vi "Complete PWM V2.vi"() -> ()   [LabVIEW 2023]
uses:
  <vilib>/Utility/error.llb/DialogType.ctl
  <vilib>/DAQmx/write.llb/DAQmx Write (Counter Frequency 1Chan 1Samp).vi
  <vilib>/DAQmx/create/channels.llb/DAQmx Create Channel (CO-Pulse Generation-Frequency).vi
  <vilib>/DAQmx/configure/timing.llb/DAQmx Timing (Implicit).vi
  <vilib>/DAQmx/miscellaneous.llb/DAQmx Fill In Error Info.vi
panel:
  out "OUT Gate":bool
  out "IN Gate":bool
  in  "stop":bool
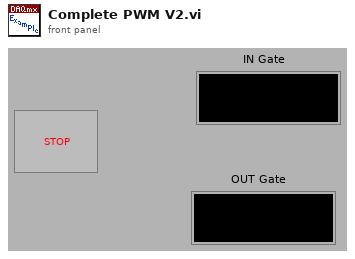
[diagram p1: front panel]
types:
  T1 = typedef "DialogType.ctl" = u16
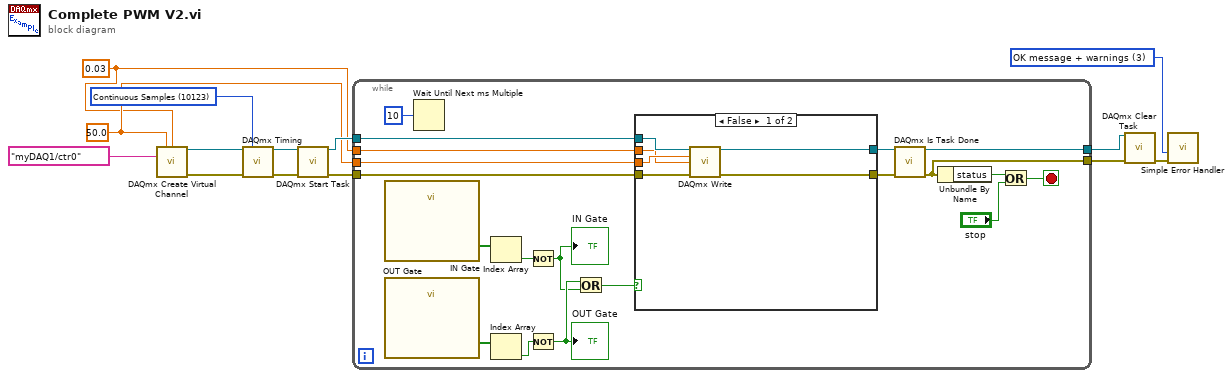
[diagram p0: block diagram]
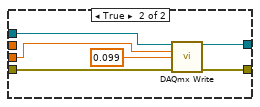
[diagram p2: hidden frame]
diagram:
  w1 = 0.03 ("Duty Cycle")
  w2 = 50.0 ("Frequency")
  w3 = T1 3 items=["no dialog", "OK message", "continue or stop message", "OK message + warnings", "continue/stop + warnings"] ("type of dialog (OK msg:1)")
  w6 = 10123 items=["Finite Samples"=10178, "Continuous Samples"=10123] ("sample mode")
  n1 = call-poly <vilib>:"DAQmx Create Virtual Channel.vi"("frequency"=w2, "duty cycle"=w1, "counter"=tag "myDAQ1/ctr0" ("Counter(s)")) -> ("task out"=w11:refnum<k21>, "error out"=w14:errorcluster)  [unwired: 11 in]
  n2 = call-poly <vilib>:"DAQmx Timing.vi"("task/channels in"=w11, "sample mode"=w6, "error in"=w14) -> ("task out"=w7:refnum<k21>, "error out"=w8:errorcluster)  [unwired: 11 in]
  n3 = call <vilib>:"DAQmx Start Task.vi"("task/channels in"=w7, "error in"=w8) -> ("task out"=w10:refnum<k21>, "error out"=w13:errorcluster)  [unwired: 12 in]
  n4 = while {
    tunnel: w13 -> [w25]
    tunnel: w10 -> [w26]
    tunnel: [w33] -> w9
    tunnel: [w32] -> w4
    tunnel: w2 -> [w24]
    tunnel: w1 -> [w15]
    stop <- w31 stop-if-true
    n5 = call "IN Gate"() -> ("data"=w22:bool[])  [unwired: 17 in, 2 out]
    n6 = call "OUT Gate"() -> ("data"=w20:bool[])  [unwired: 17 in, 2 out]
    n7 = Wait Until Next ms Multiple(millisecond multiple=u32 10) -> ()  [unwired: 1 out]
    n8 = Index Array(array=w22) -> (element=w21:bool)  [unwired: 1 in]
    n9 = Index Array(array=w20) -> (element=w19:bool)  [unwired: 1 in]
    n10 = Not(x=w21) -> (.not. x?=w16:bool)
    "IN Gate" <- w16
    n11 = Not(x=w19) -> (.not. x?=w17:bool)
    "OUT Gate" <- w17
    n12 = Or(x=w17, y=w16) -> (x .or. y?=w18:bool)
    n13 = case shown="False" w18 {
      tunnel: [w37 w45] -> w28
      tunnel: [w36 w44] -> w27
      tunnel: w26 -> [w39 w43]
      tunnel: w25 -> [w38 w42]
      tunnel: w24 -> [w35 w41]
      tunnel: w15 -> [w34 _]
      frame False {
        n14 = call-poly <vilib>:"DAQmx Write.vi"("task/channels in"=w39, "frequency"=w35, "duty cycle"=w34, "error in"=w38) -> ("task out"=w37:refnum<k21>, "error out"=w36:errorcluster)  [unwired: 9 in, 1 out]
      }
      frame True {
        n15 = call-poly <vilib>:"DAQmx Write.vi"("task/channels in"=w43, "frequency"=w41, "duty cycle"=0.099 ("Duty Cycle"), "error in"=w42) -> ("task out"=w45:refnum<k21>, "error out"=w44:errorcluster)  [unwired: 9 in, 1 out]
      }
    }
    n16 = call <vilib>:"DAQmx Is Task Done.vi"("task/channels in"=w28, "error in"=w27) -> ("task out"=w33:refnum<k21>, "error out"=w32:errorcluster)  [unwired: 11 in, 1 out]
    n17 = Unbundle By Name(w32) -> ("status"=w30:bool)
    n18 = Or(x=w30, y="stop") -> (x .or. y?=w31:bool)
  }
  n19 = call <vilib>:"DAQmx Clear Task.vi"("task in"=w9, "error in"=w4) -> ("error out"=w12:errorcluster)  [unwired: 13 in]
  n20 = call <vilib>:"Simple Error Handler.vi"("type of dialog (OK msg:1)"=w3, "error in (no error)"=w12) -> ()  [unwired: 3 in, 5 out]
